vi "Drive from Recorded File.vi"(11 "Recorded Filename":T1(ring)) -> ()   [LabVIEW 2019]
uses:
  <vilib>/Utility/file.llb/Read Delimited Spreadsheet (DBL).vi
  <vilib>/Rock Robotics/Network Tables/NT Write Number.vi
panel:
  out "all rows":dbl[][](array[numeric])
  out "array w/ subset deleted":dbl[][](array[numeric])
  out "Speed":dbl[](array[numeric])
  out "Turn":dbl[](array[numeric])
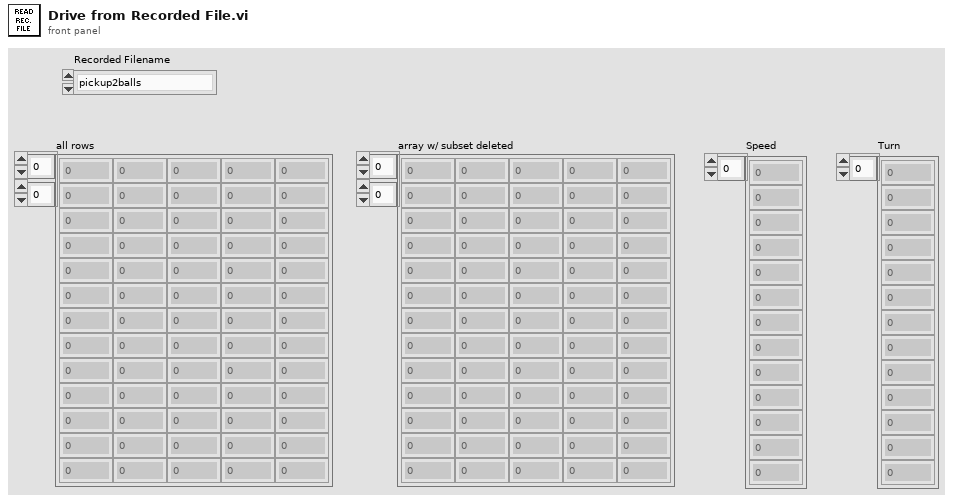
[diagram p1: front panel]
types:
  T1 = enum16{"pickup2balls", "drivetoshoot", "pickup5balls", "drivetoshoot5balls"}
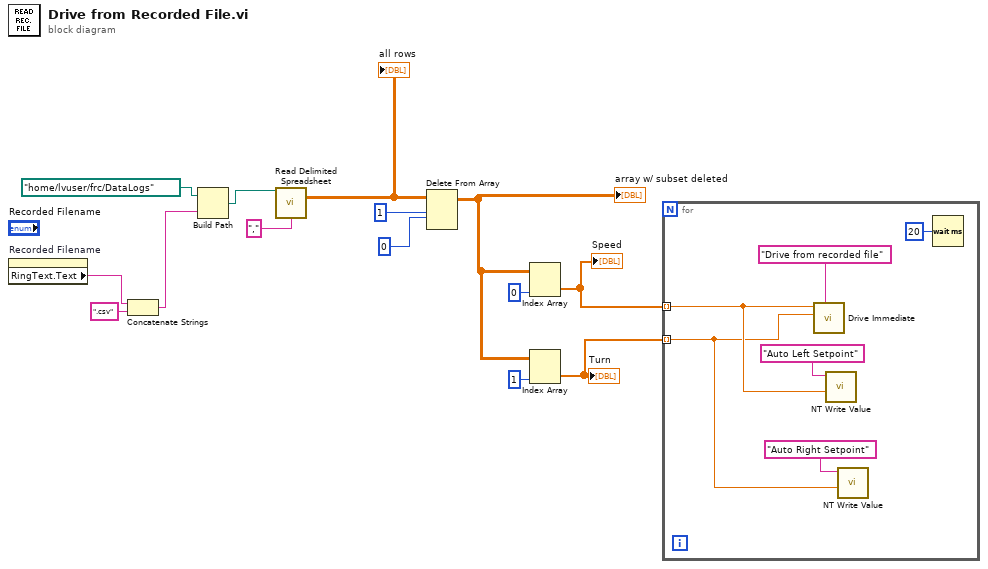
[diagram p0: block diagram]
diagram:
  n1 = property on="Recorded Filename" class="Enum (strict)"() -> ("RingText.Text"=w2:string)  [unwired: 2 in, 2 out]
  n2 = Concatenate Strings(w2, ".csv" ("string")) -> (w1:string)
  n3 = Build Path(base path=path "/home/lvuser/frc/DataLogs", name or relative path=w1) -> (appended path=w4:path)
  n4 = call-poly <vilib>:"Read Delimited Spreadsheet.vi"("file path (dialog if empty)"=w4, "delimiter (\\t)"="," ("delimiter (\\t)")) -> ("all rows"=w9:dbl[][])  [unwired: 8 in, 5 out]
  "all rows" <- w9
  n5 = Delete From Array(array=w9, length=1, index (row)=0) -> (array with subset deleted=w14:dbl[][])  [unwired: 1 in, 1 out]
  "array w/ subset deleted" <- w14
  n6 = Index Array(array=w14, index (col)=0 ("disabled index (col)")) -> (element=w7:dbl[])  [unwired: 1 in]
  "Speed" <- w7
  n7 = Index Array(array=w14, index (col)=1 ("disabled index (col)")) -> (element=w6:dbl[])  [unwired: 1 in]
  "Turn" <- w6
  n8 = for {
    tunnel: w7 -> [w16] mode=indexing
    tunnel: w6 -> [w15] mode=indexing
    n9 = call "Drive Immediate.vi"("Description"="Drive from recorded file", "Right Setpoint"=w15, "Left Setpoint"=w16) -> ()  [unwired: 8 in, 1 out]
    n10 = call-poly <vilib>:"NT Write Value.vi"("Numeric"=w16, "Name"="Auto Left Setpoint") -> ()  [unwired: 9 in, 1 out]
    n11 = call-poly <vilib>:"NT Write Value.vi"("Numeric"=w15, "Name"="Auto Right Setpoint") -> ()  [unwired: 9 in, 1 out]
    n12 = Wait (ms)(milliseconds to wait=u32 20) -> ()  [unwired: 1 out]
  }
